vi "svx_SC Line Display Marker.vi"(4 "Marker Style":u8, 6 "Marker Color":u32, 7 "time/rev/RPM":string, 8 "Cursor.Visible":bool, 9 "Marker Values":dbl[](array[numeric]), 10 "Marker Position":cluster{dbl, dbl}[](array[cluster]), 11 "Shaft Centerline":refnum<vi>) -> ()   [LabVIEW 2017, in "SVX SC Line.xctl"]
uses:
  <vilib>/addons/_XControls/Shaft Centerline/SVX SC Line.xctl
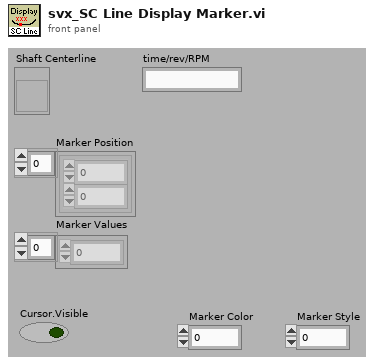
[diagram p1: front panel]
types:
  T1 = cluster{"Name":string, "Color":u32, "Style":u8, "Point Style":u8, "Name Visible":bool, "Allow Drag":bool, "Annotation Mode":u32, "Plot":i32, "Index":i32, "Position":cluster{"X":dbl, "Y":dbl}, "X Scale":u32, "Y Scale":u32, "Show Arrow":bool, "Lock Name":bool, "Plot Area":i32, "Label Offset":cluster{"X":dbl, "Y":dbl}}
  T2 = cluster{"Name":string, "Color":u32, "Style":u8, "Point Style":u8, "Name Visible":bool, "Allow Drag":bool, "Annotation Mode":u32, "Plot":i32, "Index":i32, "Position":cluster{"X":dbl, "Y":dbl}, "X Scale":u32, "Y Scale":u32, "Show Arrow":bool, "Lock Name":bool, "Plot Area":i32, "Label Offset":cluster{"X":dbl, "Y":dbl}}[]
  T3 = typedef "LVAnnotationListTypeDef.ctl" = cluster{"Name":string, "Color":u32, "Style":u8, "Point Style":u8, "Name Visible":bool, "Allow Drag":bool, "Annotation Mode":u32, "Plot":i32, "Index":i32, "Position":cluster{"X":dbl, "Y":dbl}, "X Scale":u32, "Y Scale":u32, "Show Arrow":bool, "Lock Name":bool, "Plot Area":i32, "Label Offset":cluster{"X":dbl, "Y":dbl}}[]
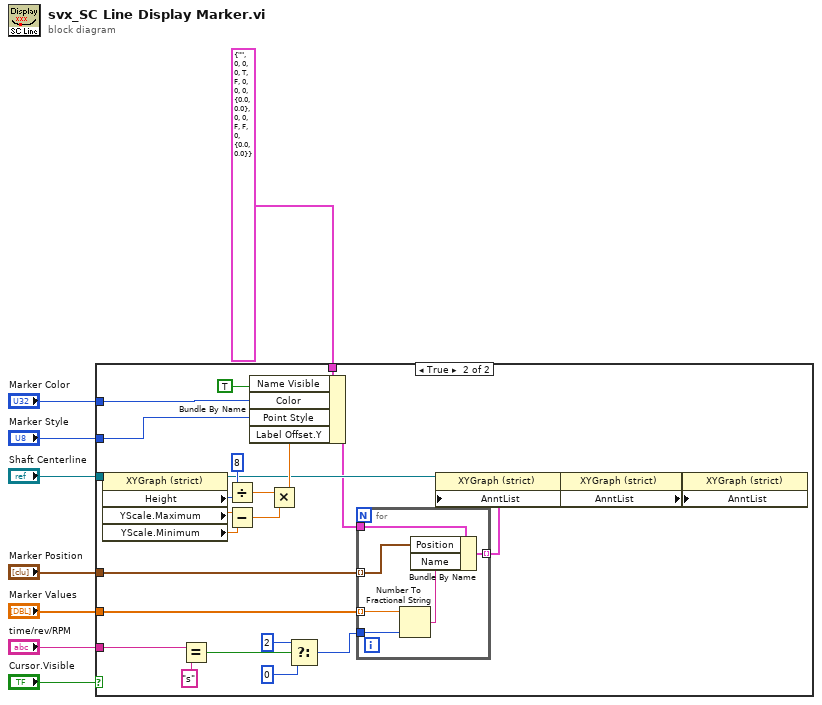
[diagram p0: block diagram]
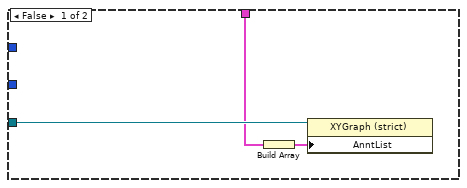
[diagram p2: hidden frame]
diagram:
  n1 = case shown="True" "Cursor.Visible" {
    tunnel: "Marker Values" -> [_ w37]
    tunnel: "Marker Position" -> [_ w25]
    tunnel: "Marker Color" -> [_ w36]
    tunnel: "Marker Style" -> [_ w35]
    tunnel: "time/rev/RPM" -> [_ w20]
    tunnel: "Shaft Centerline" -> [w11 w34]
    tunnel: T1 {"Name"="", "Color"=0, "Style"=0, "Point Style"=0, "Name Visible"=TRUE, "Allow Drag"=FALSE, "Annotation Mode"=0, "Plot"=0, "Index"=0, "Position"={"X"=0.0, "Y"=0.0}, "X Scale"=0, "Y Scale"=0, "Show Arrow"=FALSE, "Lock Name"=FALSE, "Plot Area"=0, "Label Offset"={"X"=0.0, "Y"=0.0}} ("element") -> [w10 w26]
    frame False {
      n2 = Build Array(w10) -> (w9:T2)
      n3 = property class="XYGraph (strict)"(reference=w11, "AnntList"=w9) -> ()  [unwired: 1 in, 2 out]
    }
    frame True {
      n4 = property class="XYGraph (strict)"(reference=w34) -> (reference out=w17:refnum<vi>, "Height"=w33:u32, "YScale.Maximum"=w31:dbl, "YScale.Minimum"=w30:dbl)  [unwired: 1 in, 1 out]
      n5 = Equal?(x=w20, y="s") -> (x = y?=w19:bool)
      n6 = Divide(x=u32 8, y=w33) -> (x/y=w29:dbl)
      n7 = Subtract(x=w31, y=w30) -> (x-y=w28:dbl)
      n8 = Multiply(x=w29, y=w28) -> (x*y=w27:dbl)
      n9 = Bundle By Name(cluster=w26, "Name Visible"=TRUE, "Color"=w36, "Point Style"=w35, "Label Offset.Y"=w27) -> (w16:T1)
      n10 = Select(t=i16 2 ("precision (6)"), s=w19, f=i16 0 ("precision (6)")) -> (s? t:f=w22:i16)
      n11 = for {
        tunnel: w37 -> [w43] mode=indexing
        tunnel: w22 -> [w42]
        tunnel: w25 -> [w40] mode=indexing
        tunnel: w16 -> [w41]
        tunnel: [w38] -> w15 mode=indexing
        n12 = Number To Fractional String(number=w43, precision (6)=w42) -> (F-format string=w39:string)  [unwired: 2 in]
        n13 = Bundle By Name(cluster=w41, "Position"=w40, "Name"=w39) -> (w38:T1)
      }
      n14 = property class="XYGraph (strict)"(reference=w17, "AnntList"=w15) -> (reference out=w14:refnum<vi>)  [unwired: 1 in, 1 out]
      n15 = property class="XYGraph (strict)"(reference=w14) -> (reference out=w13:refnum<vi>, "AnntList"=w12:T3)  [unwired: 1 in, 1 out]
      n16 = property class="XYGraph (strict)"(reference=w13, "AnntList"=w12) -> ()  [unwired: 1 in, 2 out]
    }
  }
